vi "Format VI Information - Folder Report.vi"(0 "file":path[](array[path]), 11 "error in":errorcluster) -> (4 "output files path":path, 6 "per file report string":string, 15 "error out":errorcluster)   [LabVIEW 2019, in "MD Generator.lvlib"]
uses:
  MD Generator.lvlib
  Filter.ctl
panel:
  in  "image directory":path
  in  "html directory":path
  in  "md directory":path
  in  "filter for":T1
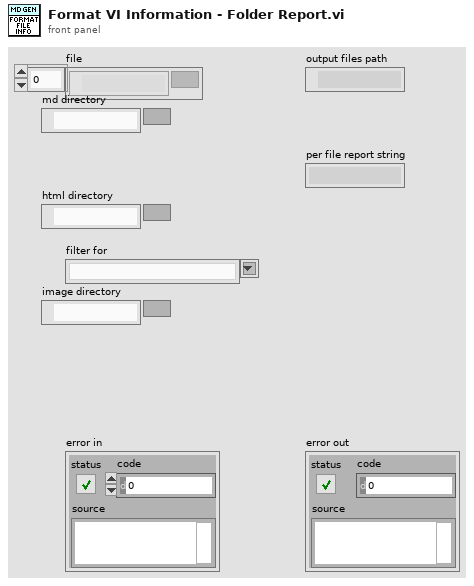
[diagram p1: front panel]
types:
  T1 = typedef "MD Generator.lvlib/Filter.ctl" = string
  T2 = enum32{"Custom", "Standard", "Using Panel", "Using SubVI", "Complete"}
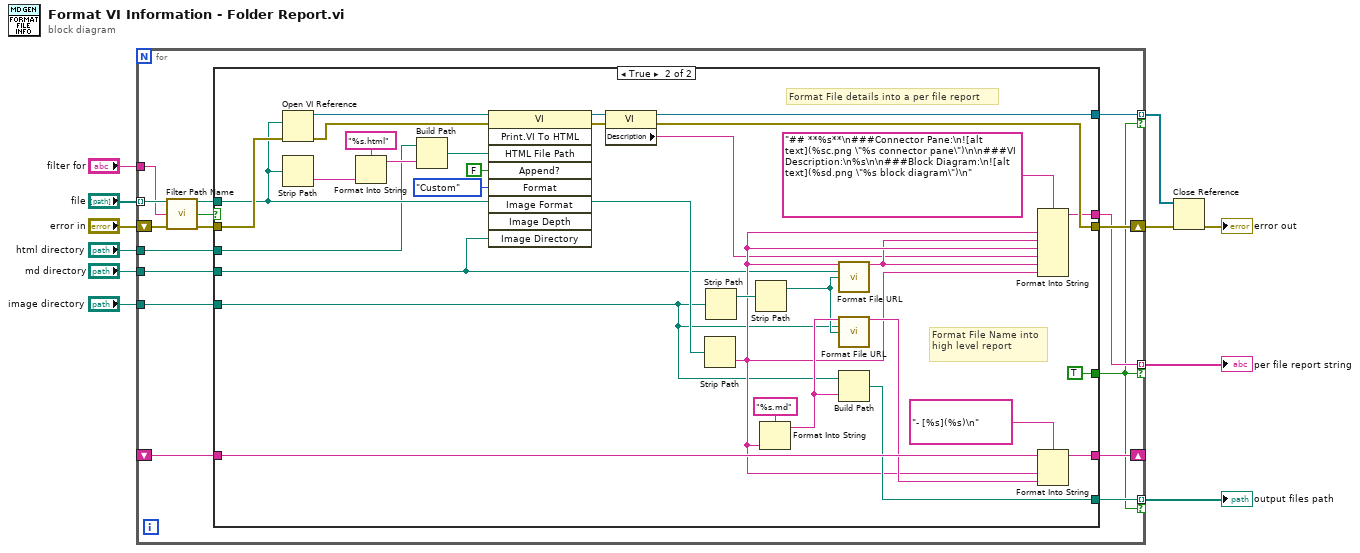
[diagram p0: block diagram]
diagram:
  n1 = for {
    tunnel: "file" -> [w29] mode=indexing
    tunnel: [w21] -> w4 mode=indexing if=w17
    shift-right: [w24] -> w12
    shift-left: "error in" -> [w28]
    tunnel: "filter for" -> [w27]
    tunnel: [w19] -> w13 mode=indexing if=w17
    shift-right: [w22] -> w6
    shift-left: [w23] -> w7
    tunnel: [w20] -> w5 mode=indexing if=w17
    tunnel: "image directory" -> [w16]
    tunnel: "html directory" -> [w15]
    tunnel: "md directory" -> [w14]
    n2 = call "Filter Path Name.vi"("file or directory paths"=w29, "filter for"=w27, "error in"=w28) -> ("matched file paths"=w25:path, "matched"=w18:bool, "error out"=w26:errorcluster)  [unwired: 10 in]
    n3 = case shown="True" w18 {
      tunnel: w26 -> [w31 w62]
      tunnel: w25 -> [_ w61]
      tunnel: [w31 w63] -> w24
      tunnel: w23 -> [w30 w60]
      tunnel: [w30 w59] -> w22
      tunnel: [_ w58] -> w21
      tunnel: [_ w51] -> w20
      tunnel: [_ w50] -> w19
      tunnel: [_ TRUE] -> w17
      tunnel: w16 -> [_ w34]
      tunnel: w15 -> [_ w33]
      tunnel: w14 -> [_ w32]
      frame False {
      }
      frame True {
        # "Format File details into a per file report"
        # "Format File Name into high level report"
        n4 = Open VI Reference(vi path=w61, error in (no error)=w62) -> (vi reference=w47:refnum<vi>, error out=w49:errorcluster)  [unwired: 4 in]
        n5 = Strip Path(path=w61) -> (name=w40:string)  [unwired: 1 out]
        n6 = Format Into String(format string="%s.html", w40) -> (resulting string=w42:string)  [unwired: 2 in, 1 out]
        n7 = Build Path(base path=w33, name or relative path=w42) -> (appended path=w43:path)
        n8 = invoke class="VI" method="Print.VI To HTML"(reference=w47, error in=w49, "HTML File Path"=w43, "Append?"=FALSE, "Format"=T2."Custom", "Image Directory"=w32) -> (reference out=w46:refnum<vi>, error out=w48:errorcluster)  [unwired: 3 in, 7 out]
        n9 = property class="VI"(reference=w46, error in=w48) -> (reference out=w50:refnum<vi>, error out=w63:errorcluster, "Description"=w35:string)
        n10 = Strip Path(path=w61) -> (name=w37:string)  [unwired: 1 out]
        n11 = Strip Path(path=w34) -> (stripped path=w52:path)  [unwired: 1 out]
        n12 = Strip Path(path=w52) -> (stripped path=w38:path)  [unwired: 1 out]
        n13 = Format Into String(format string="%s.md", w37) -> (resulting string=w54:string)  [unwired: 2 in, 1 out]
        n14 = call "Format File URL.vi"("file name"=w37, "file dir"=w32, "base dir"=w38) -> ("image URL string"=w36:string)  [unwired: 12 in]
        n15 = call "Format File URL.vi"("file name"=w54, "file dir"=w34, "base dir"=w38) -> ("image URL string"=w53:string)  [unwired: 12 in]
        n16 = Build Path(base path=w34, name or relative path=w54) -> (appended path=w51:path)
        n17 = Format Into String(format string="## **%s**\n###Connector Pane:\n![alt text](%sc.png \"%s connector pane\")\n\n###VI Description:\n%s\n\n###Block Diagram:\n![alt text](%sd.png \"%s block diagram\")\n", w37, w36, w37, w35, w36, w37) -> (resulting string=w58:string)  [unwired: 2 in, 1 out]
        n18 = Format Into String(format string="- [%s](%s)\n", initial string=w60, w37, w53) -> (resulting string=w59:string)  [unwired: 1 in, 1 out]
      }
    }
  }
  "output files path" <- w5
  "per file report string" <- w4
  n19 = Close Reference(reference=w13, error in (no error)=w12) -> (error out=→"error out":errorcluster)
